vi "arduino tres.vi"() -> ()   [LabVIEW 2013]
uses:
  <vilib>/LabVIEW Interface for Arduino/Type Defs/Board Type.ctl
  <vilib>/LabVIEW Interface for Arduino/Type Defs/Connection Type.ctl
  <vilib>/LabVIEW Interface for Arduino/Type Defs/Pin Mode.ctl
  <vilib>/LabVIEW Interface for Arduino/LabVIEW Interface for Arduino.lvlib
panel:
  out "ENTRADA":dbl
  in  "stop":bool
  out "LED":bool
  in  "Pin Mode (Input)":T1
  in  "Digital I/O Pin":u8
  in  "Connection Type (USB/Serial)":T2
  in  "Board Type (Uno)":T3
  in  "Baud Rate (115200)":u32=115200
  in  "VISA resource":refnum<visa-resource-name>
  # "UNIVERSIDAD DE CUNDINAMARCA\nINGENIERIA DE SISTEMAS\nELECTIVA PROFESIONAL IV\nANDY CAMARGO\nRAFAEL REYES\nSEMESTRE X\nEXTENCION CHIA"
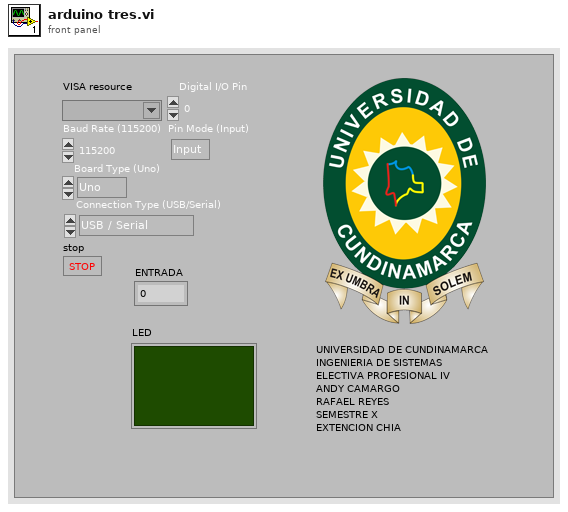
[diagram p1: front panel]
types:
  T1 = typedef "LabVIEW Interface for Arduino.lvlib/Pin Mode.ctl" = enum8{"Input", "Output"}
  T2 = typedef "LabVIEW Interface for Arduino.lvlib/Connection Type.ctl" = enum8{"USB / Serial", "XBEE", "BlueSmirf (Bluetooth)"}
  T3 = typedef "LabVIEW Interface for Arduino.lvlib/Board Type.ctl" = enum16{"Uno", "Dimuelanove w/Atmega 328", "Mega 2560"}
  T4 = typedef "LabVIEW Interface for Arduino.lvlib/Arduino Resource.ctl" = cluster{"VISA resource":refnum<visa-resource-name>, "Board Type":T3, "Connection Type":enum8{"USB / Serial"}, "Bytes Per Packet (15)":u8}
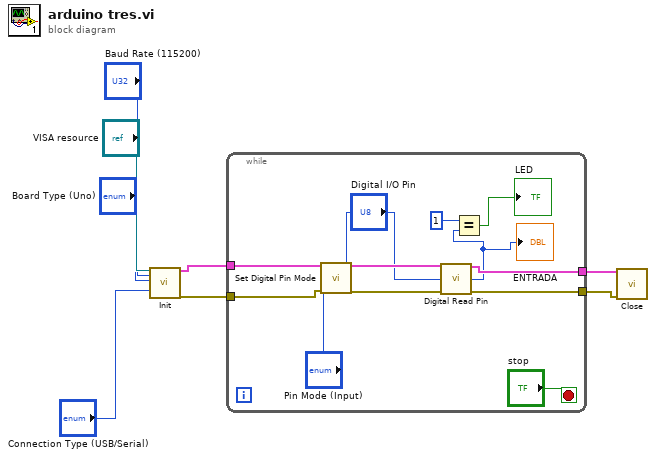
[diagram p0: block diagram]
diagram:
  n1 = call <vilib>:"Init.vi"("VISA resource"="VISA resource", "Baud Rate (115200)"="Baud Rate (115200)", "Board Type (Uno)"="Board Type (Uno)", "Connection Type (USB/Serial)"="Connection Type (USB/Serial)") -> ("Arduino Resource"=w8:T4, "error out"=w5:errorcluster)  [unwired: 14 in]
  n2 = while {
    tunnel: w8 -> [w20]
    tunnel: [w18] -> w7
    tunnel: [w17] -> w6
    tunnel: w5 -> [w15]
    stop <- "stop" stop-if-true
    n3 = call <vilib>:"Set Digital Pin Mode.vi"("Arduino Resource"=w20, "Digital I/O Pin"="Digital I/O Pin", "Pin Mode (Input)"="Pin Mode (Input)", "error in"=w15) -> ("Arduino Resource"=w19:T4, "error out"=w16:errorcluster)  [unwired: 10 in]
    n4 = call <vilib>:"Digital Read Pin.vi"("Arduino Resource"=w19, "Digital I/O Pin (0)"="Digital I/O Pin", "error in"=w16) -> ("Arduino Resource"=w18:T4, "Value"=w9:u8, "error out"=w17:errorcluster)  [unwired: 10 in]
    "ENTRADA" <- w9
    n5 = Equal?(x=u8 1, y=w9) -> (x = y?=→"LED":bool)
  }
  n6 = call <vilib>:"Close.vi"("Arduino Resource"=w7, "error in"=w6) -> ()  [unwired: 13 in, 1 out]
